vi "Select FPGA.vi"(8 "error in":errorcluster, 11 "Item Ref in":T3 format="%.0x") -> (0 "error out":errorcluster, 1 "FPGA Info":T1, 2 "FPGA Reference":T3=18446744073709551615 format="%.0x", 3 "Item Ref out":T3 format="%.0x", 4 "Cancelled?":bool, 5 "VS FPGA?":bool, 7 "Bitfile Path out":path)   [LabVIEW 2012, in "AIT 429 System Explorer.lvlib"]
uses:
  AIT 429 System Explorer.lvlib
  <vilib>/NI Veristand/Custom Device API/Custom Device Item Ref.ctl
  <userlib>/_FPGA Interface Advanced Tools/FPGA Bitfile Utility/TypeDefs/Scalar Register Set.ctl
  <userlib>/_FPGA Interface Advanced Tools/FPGA Bitfile Utility/TypeDefs/Scalar Register.ctl
  <vilib>/rvi/Utilities/XML/nirviXML_GetValue.vi
  <vilib>/rvi/Utilities/XML/nirviXML_GetValue_String.vi
  <vilib>/NI Veristand/Custom Device Tools/Custom Device Utility Library/Custom Device Utility Library.lvlib
  <vilib>/NI Veristand/Custom Device API/Custom Device API.lvlib
  <userlib>/_FPGA Interface Advanced Tools/FPGA Bitfile Utility/FPGA Bitfile Utility.lvlib
panel:
  in  "Bitfile Path":path
  in  "Cancel":bool
  in  "FPGA Selection Type":T2(radio)
  in  "OK":bool
  in  "RIO Device Address":u16(ring)
  in  "RIO Device Address":string
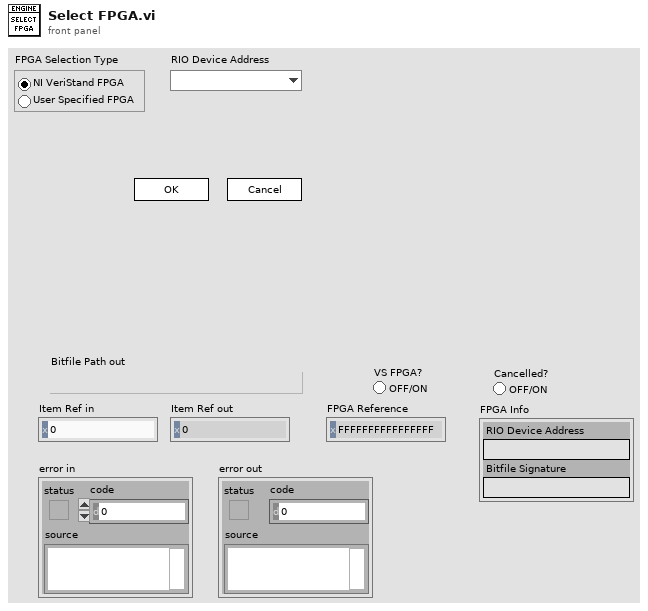
[diagram p1: front panel]
types:
  T1 = cluster{"RIO Device Address":string, "Bitfile Signature":string}
  T2 = enum32{"NI VeriStand FPGA", "User Specified FPGA"}
  T3 = typedef "Custom Device API.lvlib/Custom Device Item Ref.ctl" = u64
  T4 = typedef "FPGA Bitfile Utility.lvlib/Scalar Register Set.ctl" = cluster{"Boolean":T5[], "I8":T5[], "I16":T5[], "I32":T5[], "I64":T5[], "U8":T5[], "U16":T5[], "U32":T5[], "U64":T5[]}
  T5 = typedef "FPGA Bitfile Utility.lvlib/Scalar Register.ctl" = cluster{"Address":u32, "Name":string}
  T6 = cluster{"MD5":string, "Indicator Scalars":T4, "Control Scalars":T4}[]
  T7 = enum8{"Enabled", "Disabled", "Disabled and Grayed Out"}
  T8 = cluster{"MD5":string, "Indicator Scalars":T4, "Control Scalars":T4}
  T9 = typedef "Custom Device API.lvlib/Custom Device Item Info.ctl" = cluster{"Name":string, "Is Channel":bool, "GUID":string, "Is Waveform":bool}
  T10 = cluster{"Bitfile Signature":string, "Indicator Scalars":T4, "Control Scalars":T4}
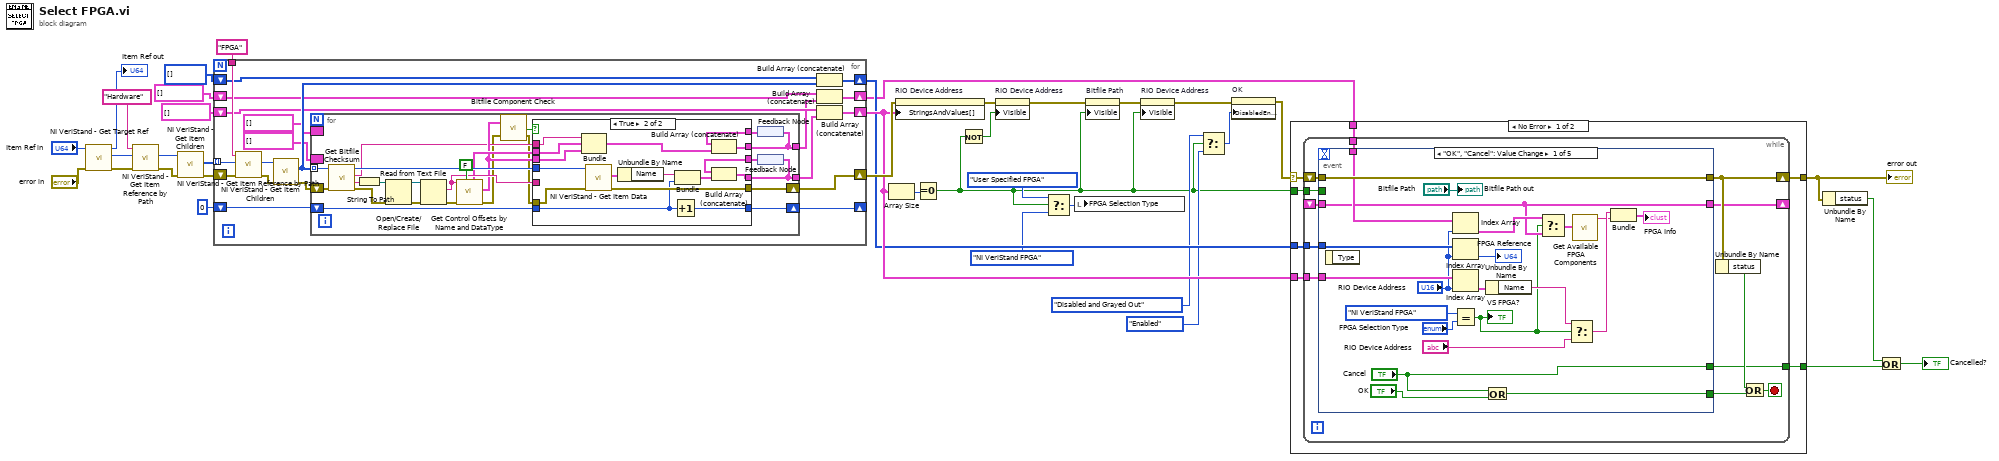
[diagram p0: block diagram]
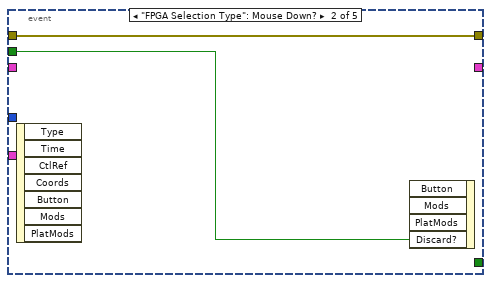
[diagram p2: hidden frame]
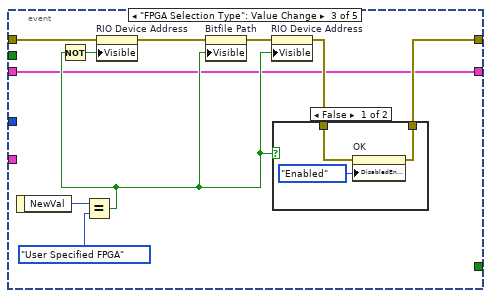
[diagram p3: hidden frame]
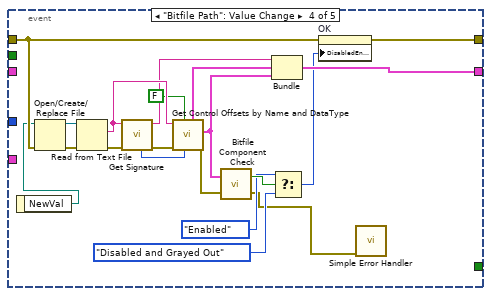
[diagram p5: hidden frame]
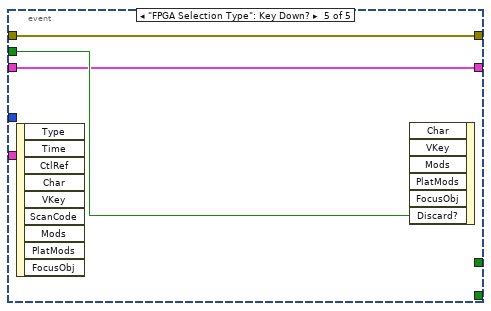
[diagram p6: hidden frame]
diagram:
  n1 = call <vilib>:"NI VeriStand - Get Target Ref.vi"("error in"="error in", "Item Ref in"="Item Ref in") -> ("error out"=w33:errorcluster, "Target Ref"=w37:T3, "Item Ref out"=→"Item Ref out":T3)  [unwired: 6 in, 1 out]
  n2 = call <vilib>:"NI VeriStand - Get Item Reference by Path.vi"("error in (no error)"=w33, "Root Ref"=w37, "Item Path in"="Hardware") -> ("error out"=w34:errorcluster, "Item Ref"=w35:T3)  [unwired: 5 in, 2 out]
  n3 = call <vilib>:"NI VeriStand - Get Item Children.vi"("error in (no error)"=w34, "Item Ref in"=w35) -> ("error out"=w30:errorcluster, "Child Refs"=w32:T3[])  [unwired: 6 in, 2 out]
  n4 = for {
    tunnel: w32 -> [w57] mode=indexing
    tunnel: "FPGA" ("Item Path in") -> [w56]
    shift-right: [w45] -> w29
    shift-left: w30 -> [w54]
    shift-right: [w49] -> w20
    shift-left: T3[] [] -> [w48]
    shift-right: [w47] -> w21
    shift-left: cluster{"Name":string, u16}[] [] -> [w46]
    shift-right: [w44] -> _
    shift-left: u16 0 -> [w43]
    shift-right: [w41] -> w6
    shift-left: T6 [] -> [w40]
    n5 = call <vilib>:"NI VeriStand - Get Item Reference by Path.vi"("error in (no error)"=w54, "Root Ref"=w57, "Item Path in"=w56) -> ("error out"=w53:errorcluster, "Item Ref"=w55:T3)  [unwired: 5 in, 2 out]
    n6 = call <vilib>:"NI VeriStand - Get Item Children.vi"("error in (no error)"=w53, "Item Ref in"=w55) -> ("error out"=w52:errorcluster, "Child Refs"=w50:T3[])  [unwired: 6 in, 2 out]
    n7 = for {
      tunnel: w50 -> [w78] mode=indexing
      tunnel: [w64] -> w51
      shift-right: [w81] -> w45
      shift-left: w52 -> [w77]
      shift-right: [w80] -> w44
      shift-left: w43 -> [w79]
      border: cluster{"Name":string, u16}[] [] -> [_]
      border: T6 [] -> [_]
      tunnel: [w62] -> w39
      n8 = call "Get Bitfile Checksum.vi"("error in (no error)"=w77, "ID in"=w78) -> ("error out"=w73:errorcluster, "Path"=w75:string, "MD5"=w60:string, "ID out"=w76:T3)  [unwired: 6 in]
      n9 = String To Path(string=w75) -> (path=w74:path)
      n10 = Open/Create/Replace File(file path (use dialog)=w74, error in=w73) -> (refnum out=w71:refnum<file>, error out=w72:errorcluster)  [unwired: 4 in, 1 out]
      n11 = Read from Text File(file (use dialog)=w71, error in=w72) -> (text=w68:string, error out=w70:errorcluster)  [unwired: 2 in, 2 out]
      n12 = call <userlib>:"Get Control Offsets by Name and DataType.vi"("User Specified?"=FALSE, "error in"=w70, "bitfile xml in"=w68) -> ("error out"=w59:errorcluster, "Control Scalars"=w65:T4, "Indicator Scalars"=w66:T4)  [unwired: 3 in, 3 out]
      n13 = call "Bitfile Component Check.vi"("error in (no error)"=w59, "Control Scalars"=w65) -> ("error out"=w58:errorcluster, "Valid?"=w67:bool)
      n14 = feedback #1() -> (w61:T6)
      n15 = feedback #2() -> (w63:cluster{"Name":string, u16}[])
      n16 = case shown="True" w67 {
        tunnel: [w84 w99] -> w81
        tunnel: [w85 w94] -> w64
        tunnel: [w83 w97] -> w80
        tunnel: w79 -> [w83 w96]
        tunnel: w76 -> [_ w95]
        tunnel: w68 -> [_ _]
        tunnel: w58 -> [w84 w86]
        tunnel: w66 -> [_ w93]
        tunnel: w65 -> [_ w92]
        tunnel: [w82 w90] -> w62
        tunnel: w63 -> [w85 w89]
        tunnel: w61 -> [w82 w88]
        tunnel: w60 -> [_ w87]
        frame False {
        }
        frame True {
          n17 = Bundle("MD5"=w87, "Indicator Scalars"=w93, "Control Scalars"=w92) -> (w91:T8)  [unwired: 1 in]
          n18 = call <vilib>:"NI VeriStand - Get Item Data.vi"("error in (no error)"=w86, "Item Ref in"=w95) -> ("error out"=w99:errorcluster, "Item Info"=w101:T9)  [unwired: 6 in, 2 out]
          n19 = Unbundle By Name(w101) -> ("Name"=w100:string)
          n20 = Increment(x=w96) -> (x+1=w97:u16)
          n21 = Bundle("Name"=w100, w96) -> (w98:cluster{"Name":string, u16})  [unwired: 1 in]
          n22 = Build Array (concatenate)(w88, w91) -> (w90:T6)
          n23 = Build Array (concatenate)(w89, w98) -> (w94:cluster{"Name":string, u16}[])
        }
      }
      n24 = feedback-in #1(w62) -> ()
      n25 = feedback-in #2(w64) -> ()
    }
    n26 = Build Array (concatenate)(w48, w50) -> (w49:T3[])
    n27 = Build Array (concatenate)(w40, w39) -> (w41:T6)
    n28 = Build Array (concatenate)(w46, w51) -> (w47:cluster{"Name":string, u16}[])
  }
  n29 = Array Size(array=w21) -> (size(s)=w22:i32)
  n30 = property on="RIO Device Address" class="Ring (strict)"(error in=w29, "StringsAndValues[]"=w21) -> (error out=w19:errorcluster)  [unwired: 1 in, 1 out]
  n31 = Equal To 0?(x=w22) -> (x = 0?=w8:bool)
  n32 = Not(x=w8) -> (.not. x?=w18:bool)
  n33 = property on="RIO Device Address" class="Ring (strict)"(error in=w19, "Visible"=w18) -> (error out=w17:errorcluster)  [unwired: 1 in, 1 out]
  n34 = Select(t=T2."User Specified FPGA" ("x"), s=w8, f=T2."NI VeriStand FPGA" ("x")) -> (s? t:f=w15:T2)
  n35 = local write "FPGA Selection Type"(w15) -> ()
  n36 = property on="Bitfile Path" class="Path"(error in=w17, "Visible"=w8) -> (error out=w16:errorcluster)  [unwired: 1 in, 1 out]
  n37 = property on="RIO Device Address" class="Str"(error in=w16, "Visible"=w8) -> (error out=w12:errorcluster)  [unwired: 1 in, 1 out]
  n38 = Select(t=T7."Disabled and Grayed Out" ("Disabled"), s=w8, f=T7."Enabled" ("Disabled")) -> (s? t:f=w7:T7)
  n39 = property on="OK" class="Bool"(error in=w12, "DisabledEnum"=w7) -> (error out=w11:errorcluster)  [unwired: 1 in, 1 out]
  n40 = case shown="No Error" w11 {
    selector: w11 -> [w105 w182]
    tunnel: w21 -> [w108 _]
    tunnel: w20 -> [w107 _]
    tunnel: w8 -> [w106 _]
    tunnel: [w104 w182] -> w3
    tunnel: w6 -> [w103 _]
    tunnel: [w102 _] -> w4
    frame No Error {
      n41 = while {
        tunnel: w106 -> [w117]
        tunnel: w108 -> [w119]
        tunnel: w107 -> [w118]
        shift-right: [w114] -> w104
        shift-left: w105 -> [w116]
        shift-right: [w113] -> _
        shift-left: _ -> [w112]
        tunnel: w103 -> [w111]
        tunnel: [w109] -> w102
        stop <- w115 stop-if-true
        n42 = event shown="[0] \"OK\", \"Cancel\": Value Change" {
          selector: _ -> [_ _ _ _ _]
          dyn-events: _ -> [_ _ _ _ _]
          timeout: _ -> [_ _ _ _ _]
          tunnel: [w141 _ _ _ _] -> w120
          tunnel: w119 -> [w139 _ _ _ _]
          tunnel: w118 -> [w133 _ _ _ _]
          tunnel: w117 -> [_ w144 _ _ w181]
          tunnel: w116 -> [w131 w143 w152 w168 w180]
          tunnel: [w131 w143 w148 w169 w180] -> w114
          tunnel: [w127 _ w145 w167 w179] -> w113
          tunnel: w112 -> [w127 _ w145 _ w179]
          tunnel: w111 -> [w129 _ _ _ _]
          tunnel: ["Cancel" _ _ _ _] -> w109
          event "OK", "Cancel": Value Change {
            n43 = event-data() -> ()  [unwired: 1 in, 1 out]
            n44 = Index Array(array=w129, index="RIO Device Address") -> (element=w128:T8)
            n45 = Index Array(array=w133, index="RIO Device Address") -> (element=→"FPGA Reference":T3)
            n46 = Index Array(array=w139, index="RIO Device Address") -> (element=w138:cluster{"Name":string, u16})
            n47 = Equal?(x=T2."NI VeriStand FPGA", y="FPGA Selection Type") -> (x = y?=w126:bool)
            "VS FPGA?" <- w126
            n48 = Or(x="Cancel", y="OK") -> (x .or. y?=w141:bool)
            n49 = Unbundle By Name(w138) -> ("Name"=w137:string)
            n50 = Select(t=w128, s=w126, f=w127) -> (s? t:f=w125:T10)
            n51 = Select(t=w137, s=w126, f="RIO Device Address") -> (s? t:f=w123:string)
            n52 = call "Get Available FPGA Components.vi"("Register Info"=w125) -> ("Bitfile Signature"=w121:string)  [unwired: 9 in, 1 out]
            n53 = Bundle("RIO Device Address"=w123, "Bitfile Signature"=w121) -> (→"FPGA Info":T1)  [unwired: 1 in]
            "Bitfile Path out" <- "Bitfile Path"
          }
          event "FPGA Selection Type": Mouse Down? {
            n54 = event-data() -> ()  [unwired: 1 in, 7 out]
            n55 = event-data("Discard?"=w144) -> ()  [unwired: 4 in, 1 out]
          }
          event "FPGA Selection Type": Value Change {
            n56 = event-data() -> ("NewVal"=w151:T2)  [unwired: 1 in]
            n57 = Equal?(x=w151, y=T2."User Specified FPGA" ("x")) -> (x = y?=w146:bool)
            n58 = Not(x=w146) -> (.not. x?=w149:bool)
            n59 = property on="RIO Device Address" class="Ring (strict)"(error in=w152, "Visible"=w149) -> (error out=w153:errorcluster)  [unwired: 1 in, 1 out]
            n60 = property on="Bitfile Path" class="Path"(error in=w153, "Visible"=w146) -> (error out=w154:errorcluster)  [unwired: 1 in, 1 out]
            n61 = property on="RIO Device Address" class="Str"(error in=w154, "Visible"=w146) -> (error out=w147:errorcluster)  [unwired: 1 in, 1 out]
            n62 = case shown="False" w146 {
              tunnel: [w157 w158] -> w148
              tunnel: w147 -> [w156 w158]
              frame False {
                n63 = property on="OK" class="Bool"(error in=w156, "DisabledEnum"=T7."Enabled" ("Disabled")) -> (error out=w157:errorcluster)  [unwired: 1 in, 1 out]
              }
              frame True {
              }
            }
          }
          event "Bitfile Path": Value Change {
            n64 = event-data() -> ("NewVal"=w162:path)  [unwired: 1 in]
            n65 = Open/Create/Replace File(file path (use dialog)=w162, error in=w168) -> (refnum out=w173:refnum<file>, error out=w174:errorcluster)  [unwired: 4 in, 1 out]
            n66 = Read from Text File(file (use dialog)=w173, error in=w174) -> (text=w176:string, error out=w175:errorcluster)  [unwired: 2 in, 2 out]
            n67 = call <userlib>:"Get Signature.vi"("error in (no error)"=w175, "bitfile xml in"=w176) -> ("error out"=w177:errorcluster, "Bitfile Signature"=w170:string, "offset past EndTag"=w178:i32)  [unwired: 7 in]
            n68 = call <userlib>:"Get Control Offsets by Name and DataType.vi"("offset"=w178, "User Specified?"=FALSE, "error in"=w177, "bitfile xml in"=w176) -> ("error out"=w160:errorcluster, "Control Scalars"=w172:T4, "Indicator Scalars"=w171:T4)  [unwired: 2 in, 3 out]
            n69 = call "Bitfile Component Check.vi"("error in (no error)"=w160, "Control Scalars"=w172) -> ("error out"=w159:errorcluster, "Valid?"=w166:bool)
            n70 = Bundle("Bitfile Signature"=w170, "Indicator Scalars"=w171, "Control Scalars"=w172) -> (w167:T10)  [unwired: 1 in]
            n71 = Select(t=T7."Enabled" ("Disabled"), s=w166, f=T7."Disabled and Grayed Out" ("Disabled")) -> (s? t:f=w163:T7)
            n72 = property on="OK" class="Bool"(error in=w168, "DisabledEnum"=w163) -> (error out=w169:errorcluster)  [unwired: 1 in, 1 out]
            n73 = call <vilib>:"Simple Error Handler.vi"("error in (no error)"=w159) -> ()  [unwired: 4 in, 5 out]
          }
          event "FPGA Selection Type": Key Down? {
            n74 = event-data() -> ()  [unwired: 1 in, 9 out]
            n75 = event-data("Discard?"=w181) -> ()  [unwired: 6 in, 1 out]
          }
        }
        n76 = Unbundle By Name(w114) -> ("status"=w110:bool)
        n77 = Or(x=w110, y=w120) -> (x .or. y?=w115:bool)
      }
    }
    frame Error {
    }
  }
  "error out" <- w3
  n78 = Unbundle By Name(w3) -> ("status"=w2:bool)
  n79 = Or(x=w2, y=w4) -> (x .or. y?=→"Cancelled?":bool)
